vi "ChromaticAdaptation.vi"() -> ()   [LabVIEW 2011]
uses:
  <vilib>/Analysis/Matrix/Datatypes/RealMatrix.ctl
  <vilib>/Utility/file.llb/Read From Spreadsheet File (string).vi
  <vilib>/Utility/file.llb/Read From Spreadsheet File (DBL).vi
  <vilib>/Analysis/baseanly.llb/Real Inverse Matrix.vi
  <vilib>/Analysis/baseanly.llb/A x Vector.vi
  <vilib>/Analysis/Matrix/Numeric/Multiply/Multiply - RM,RM.vi
  <vilib>/Utility/file.llb/Write To Spreadsheet File (DBL).vi
  <vilib>/Analysis/NI_AALBase.lvlib
  <vilib>/Analysis/Matrix/NI_Matrix.lvlib
panel:
  in  "Close 2":bool
  in  "XYZ source white":dbl[](array[numeric]) format="%.1f"
  in  "Source XYZ":enum32{"Radio Selection 1", "Radio Selection 2"}(radio)
  in  "Src. Illuminant":string(combo)="D65"
  in  "Destination XYZ":enum32{"Radio Selection 1", "Radio Selection 2"}(radio)
  out "Adapted XYZ":dbl[](array[numeric]) format="%.1f"
  out "Adaptation Matrix":T1 format="%#.5f"
  in  "XYZ destination white":dbl[](array[numeric]) format="%.1f"
  in  "Dst. Illuminant":string(combo)="D50"
  in  "Method":string(combo)="Bradford.txt"
  in  "Close":bool
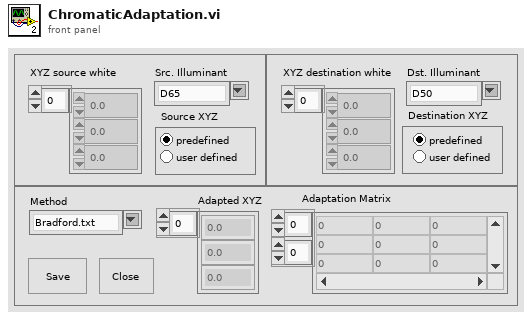
[diagram p1: front panel]
types:
  T1 = typedef "NI_Matrix.lvlib/RealMatrix.ctl" = dbl[][]
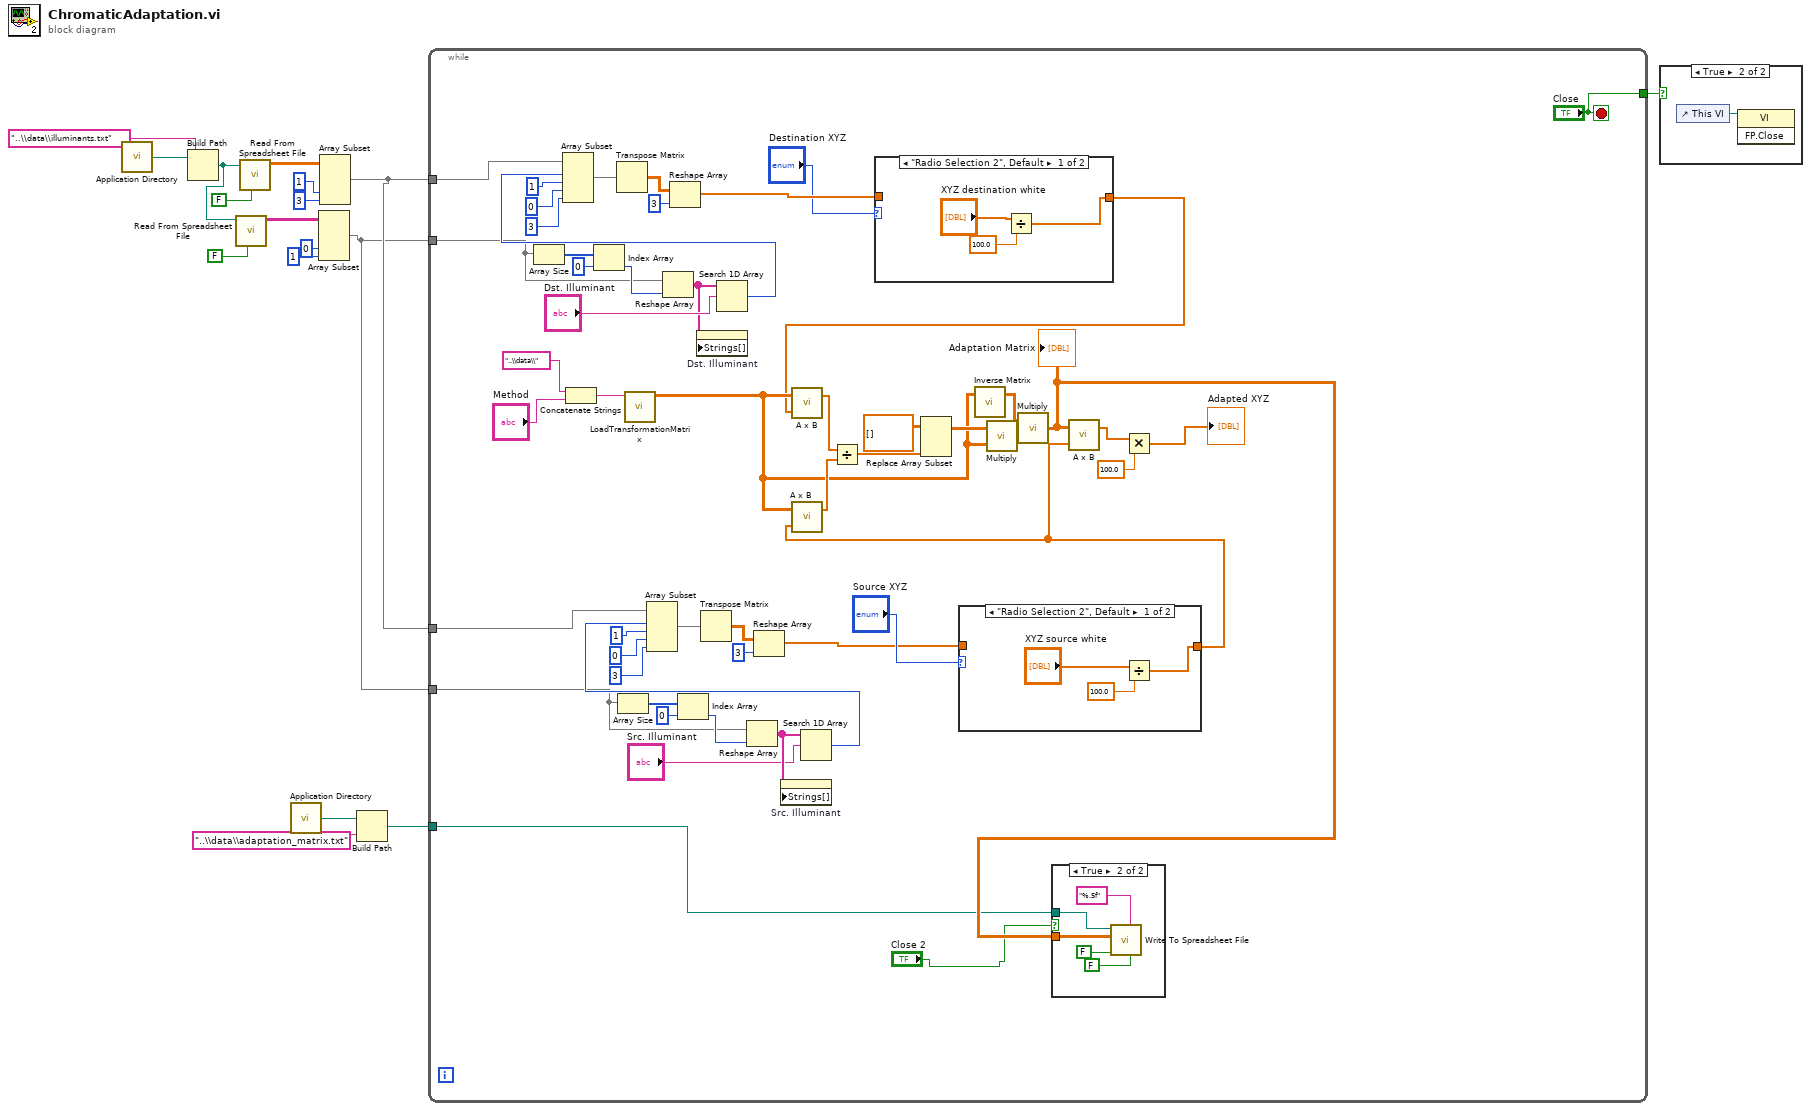
[diagram p0: block diagram]
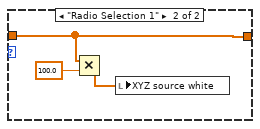
[diagram p4: hidden frame]
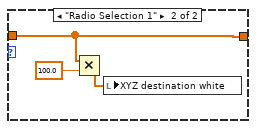
[diagram p5: hidden frame]
diagram:
  n1 = call <vilib>:"Application Directory.vi"() -> ("Application Directory"=w7:path)
  n2 = Build Path(base path=w7, name or relative path="..\\data\\illuminants.txt") -> (appended path=w12:path)
  n3 = call-poly <vilib>:"Read From Spreadsheet File.vi"("transpose (no:F)"=FALSE, "file path (dialog if empty)"=w12) -> ("all rows"=w13:string[][])  [unwired: 5 in, 4 out]
  n4 = call-poly <vilib>:"Read From Spreadsheet File.vi"("transpose (no:F)"=FALSE, "file path (dialog if empty)"=w12) -> ("all rows"=w16:dbl[][])  [unwired: 5 in, 4 out]
  n5 = call <vilib>:"Application Directory.vi"() -> ("Application Directory"=w2:path)
  n6 = Array Subset(array=w13, index (col)=0 ("index"), length (col)=1 ("length")) -> (w4:string[][])  [unwired: 2 in]
  n7 = Array Subset(array=w16, index (col)=1 ("index"), length (col)=3 ("length")) -> (w5:dbl[][])  [unwired: 2 in]
  n8 = Build Path(base path=w2, name or relative path="..\\data\\adaptation_matrix.txt") -> (appended path=w1:path)
  n9 = while {
    tunnel: ["Close"] -> w17
    tunnel: w4 -> [w52]
    tunnel: w5 -> [w54]
    tunnel: w5 -> [w26]
    tunnel: w4 -> [w25]
    tunnel: w1 -> [w20]
    stop <- "Close" stop-if-true
    n10 = Array Size(array=w52) -> (size(s)=w57:i32[])
    n11 = Concatenate Strings("..\\data\\" ("name or relative path"), "Method") -> (w68:string)
    n12 = Index Array(array=w57, index=0) -> (element=w55:i32)
    n13 = Array Size(array=w25) -> (size(s)=w36:i32[])
    n14 = call "LoadTransformationMatrix.vi"("relative path"=w68) -> ("transformation matrix"=w45:T1)  [unwired: 10 in]
    n15 = Reshape Array(w52, w55) -> (w64:string[])
    n16 = Index Array(array=w36, index=0) -> (element=w38:i32)
    n17 = property on="Dst. Illuminant" class="CmbBox"("Strings[]"=w64) -> ()  [unwired: 2 in, 2 out]
    n18 = Search 1D Array(1D array=w64, element="Dst. Illuminant") -> (index of element=w53:i32)  [unwired: 1 in]
    n19 = Array Subset(array=w54, index (row)=w53, length (row)=1 ("length"), index (col)=0 ("index"), length (col)=3 ("length")) -> (w60:dbl[][])
    n20 = Transpose Matrix(1:w60) -> (0:w59:dbl[][])
    n21 = Reshape Array(w59, 3 ("dimension size")) -> (w43:dbl[])
    n22 = Reshape Array(w25, w38) -> (w29:string[])
    n23 = property on="Src. Illuminant" class="CmbBox"("Strings[]"=w29) -> ()  [unwired: 2 in, 2 out]
    n24 = Search 1D Array(1D array=w29, element="Src. Illuminant") -> (index of element=w39:i32)  [unwired: 1 in]
    n25 = Array Subset(array=w26, index (row)=w39, length (row)=1 ("length"), index (col)=0 ("index"), length (col)=3 ("length")) -> (w33:dbl[][])
    n26 = Transpose Matrix(1:w33) -> (0:w34:dbl[][])
    n27 = Reshape Array(w34, 3 ("dimension size")) -> (w40:dbl[])
    n28 = case shown="\"Radio Selection 2\", Default" "Destination XYZ" {
      tunnel: [w81 w85] -> w18
      tunnel: w43 -> [_ w85]
      frame "Radio Selection 2", Default {
        n29 = Divide(x="XYZ destination white", y=100.0) -> (x/y=w81:dbl[])
      }
      frame "Radio Selection 1" {
        n30 = Multiply(x=w85, y=100.0) -> (x*y=w84:dbl[])
        n31 = local write "XYZ destination white"(w84) -> ()
      }
    }
    n32 = call-poly <vilib>:"A x B.vi"("Vector"=w18, "A"=w45) -> ("A x Vector"=w51:dbl[])  [unwired: 1 out]
    n33 = case shown="\"Radio Selection 2\", Default" "Source XYZ" {
      tunnel: [w75 w79] -> w27
      tunnel: w40 -> [_ w79]
      frame "Radio Selection 2", Default {
        n34 = Divide(x="XYZ source white", y=100.0) -> (x/y=w75:dbl[])
      }
      frame "Radio Selection 1" {
        n35 = Multiply(x=w79, y=100.0) -> (x*y=w78:dbl[])
        n36 = local write "XYZ source white"(w78) -> ()
      }
    }
    n37 = call-poly <vilib>:"A x B.vi"("Vector"=w27, "A"=w45) -> ("A x Vector"=w50:dbl[])  [unwired: 1 out]
    n38 = Divide(x=w51, y=w50) -> (x/y=w48:dbl[])
    n39 = Replace Array Subset(array=T1 [] ("transformation matrix"), new element=w48) -> (w47:T1)  [unwired: 2 in]
    n40 = call-poly <vilib>:"Inverse Matrix.vi"("Input Matrix"=w45) -> ("Inverse Matrix"=w44:T1)  [unwired: 1 in, 1 out]
    n41 = call-poly <vilib>:"Multiply.vi"("Real Matrix B"=w45, "Real Matrix A"=w47) -> ("A * B"=w46:T1)
    n42 = call-poly <vilib>:"Multiply.vi"("Real Matrix B"=w46, "Real Matrix A"=w44) -> ("A * B"=w21:T1)
    "Adaptation Matrix" <- w21
    n43 = case shown="True" "Close 2" {
      tunnel: w20 -> [_ w71]
      tunnel: w21 -> [_ w70]
      frame False {
      }
      frame True {
        n44 = call-poly <vilib>:"Write To Spreadsheet File.vi"("transpose? (no:F)"=FALSE, "format (%.3f)"="%.5f", "append to file? (new file:F)"=FALSE, "2D data"=w70, "file path (dialog if empty)"=w71) -> ()  [unwired: 3 in, 1 out]
      }
    }
    n45 = call-poly <vilib>:"A x B.vi"("Vector"=w27, "A"=w21) -> ("A x Vector"=w24:dbl[])  [unwired: 1 out]
    n46 = Multiply(x=w24, y=100.0) -> (x*y=→"Adapted XYZ":dbl[])
  }
  n47 = case shown="True" w17 {
    frame False {
    }
    frame True {
      n48 = control-ref of="This VI"() -> (w87:refnum<vi>)
      n49 = invoke class="VI" method="FP.Close"(reference=w87) -> ()  [unwired: 2 in, 3 out]
    }
  }
